vi "MyHostCode.vi"() -> ()   [LabVIEW 2012]
doc: "This VI was generated automatically using the FPGA Wizard. You can modify the VI normally."
uses:
  <vilib>/rvi/interface/nirviMethod/nirviMethod.xnode
  <vilib>/FPGAPlugInAG/Dynamic/niLvFpga_Run_Dynamic.vi
  <vilib>/rvi/interface/nirviCloseFPGA/nirviCloseFPGA.xnode
  <vilib>/rvi/interface/nirviOpenFPGA/nirviOpenFPGA.xnode
  <vilib>/FPGAPlugInAG/Dynamic/niLvFpga_Reset_Dynamic.vi
  MyFPGACode.vi
  <vilib>/rvi/interface/nirviReadWriteControl/nirviReadWriteControl.xnode
  <vilib>/rvi/errors/niLvFpgaAdjustHostInterfaceError.vi
  <vilib>/FPGAPlugInAG/Dynamic/niLvFpga_Close_Dynamic.vi
  NiFpgaLv.dll
  <vilib>/Utility/error.llb/Error Cluster From Error Code.vi
  <vilib>/rvi/interface/Simulation/niFpgaSimulationCallBeginRW.vi
panel:
  in  "PWM Settings (Port0/DIO5)":cluster{"ActiveTime":u32, "Period":u32}
  out "AI (ModA/AI0)":fxp<+/-,26,5> format="%.23g"
  in  "Local Stop 0":bool
  in  "Start 0":bool
  out "error out":errorcluster
  in  "Global Stop":bool
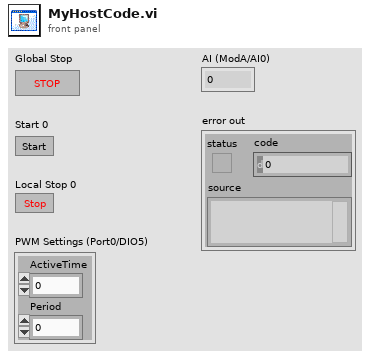
[diagram p1: front panel]
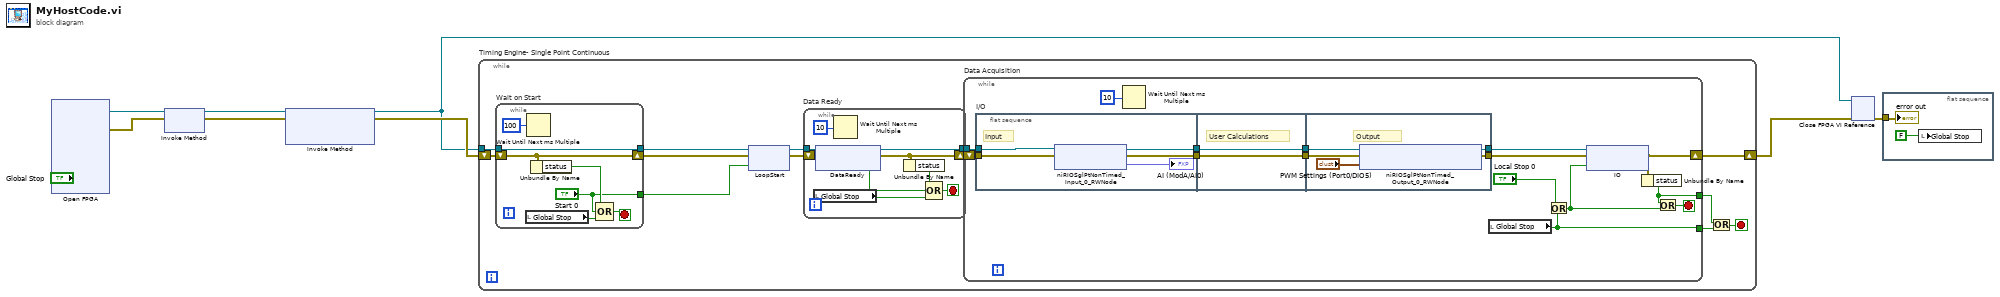
[diagram p0: block diagram]
diagram:
  n1 = xnode ("Open FPGA")() -> ("FPGA VI Reference Out"=w4:refnum<k20>, "error out"=w3:errorcluster)  [unwired: 2 in]
  n2 = xnode ("Invoke Method")("FPGA VI Reference In"=w4, "error in"=w3) -> ("FPGA VI Reference Out"=w7:refnum<k20>, "error out"=w8:errorcluster)
  n3 = xnode ("Invoke Method")("FPGA VI Reference In"=w7, "error in"=w8) -> ("FPGA VI Reference Out"=w5:refnum<k20>, "error out"=w6:errorcluster)  [unwired: 1 in]
  n4 = while "Timing Engine- Single Point Continuous" {
    tunnel: w5 -> [w20]
    shift-right: [w19] -> w2
    shift-left: w6 -> [w21]
    stop <- w14 stop-if-true
    n5 = while "Wait on Start" {
      tunnel: w20 -> [w36]
      tunnel: [w36] -> w11
      tunnel: ["Start 0"] -> w9
      shift-right: [w33] -> w10
      shift-left: w21 -> [w33]
      stop <- w37 stop-if-true
      n6 = local read "Global Stop"() -> (w34:bool)
      n7 = Wait Until Next ms Multiple(millisecond multiple=u32 100) -> ()  [unwired: 1 out]
      n8 = Unbundle By Name(w33) -> ("status"=w32:bool)
      n9 = Compound Arithmetic op=OR(w32, "Start 0", w34) -> (w37:bool)
    }
    n10 = xnode ("LoopStart")("FPGA VI Reference In"=w11, "error in"=w10, "Start 0"=w9) -> ("FPGA VI Reference Out"=w18:refnum<k20>, "error out"=w16:errorcluster)
    n11 = while "Data Ready" {
      tunnel: w18 -> [w30]
      tunnel: [w29] -> w17
      shift-right: [w23] -> w12
      shift-left: w16 -> [w28]
      stop <- w24 stop-if-true
      n12 = local read "Global Stop"() -> (w26:bool)
      n13 = xnode ("DataReady")("FPGA VI Reference In"=w30, "error in"=w28) -> ("FPGA VI Reference Out"=w29:refnum<k20>, "error out"=w23:errorcluster, "Data Ready 0"=w25:bool)
      n14 = Wait Until Next ms Multiple(millisecond multiple=u32 10) -> ()  [unwired: 1 out]
      n15 = Unbundle By Name(w23) -> ("status"=w22:bool)
      n16 = Compound Arithmetic op=OR(w22, w25, w26) -> (w24:bool)
    }
    n17 = while "Data Acquisition" {
      tunnel: w17 -> [w41]
      tunnel: [w43] -> w15
      tunnel: [w42] -> w13
      shift-right: [w44] -> w19
      shift-left: w12 -> [w40]
      stop <- w52 stop-if-true
      n18 = flat-sequence "I/O" {
        tunnel: w41 -> [w55]
        tunnel: [w56] -> w50
        tunnel: [w54] -> w47
        tunnel: w40 -> [w57]
        tunnel: w50 -> [w59]
        tunnel: [w59] -> w49
        tunnel: [w58] -> w48
        tunnel: w47 -> [w58]
        tunnel: [w63] -> w46
        tunnel: [w61] -> w45
        tunnel: w49 -> [w64]
        tunnel: w48 -> [w62]
        frame #0 {
          # "Input"
          n19 = xnode ("niRIOSglPtNonTimed_Input_0_RWNode")("FPGA VI Reference In"=w55, "error in"=w57) -> ("FPGA VI Reference Out"=w54:refnum<k20>, "error out"=w56:errorcluster, "AI (ModA/AI0)"=→"AI (ModA/AI0)":fxp<+/-,26,5>)
        }
        frame #1 {
          # "User Calculations"
        }
        frame #2 {
          # "Output"
          n20 = xnode ("niRIOSglPtNonTimed_Output_0_RWNode")("FPGA VI Reference In"=w62, "error in"=w64, "PWM Settings (Port0/DIO5)"="PWM Settings (Port0/DIO5)") -> ("FPGA VI Reference Out"=w61:refnum<k20>, "error out"=w63:errorcluster)
        }
      }
      n21 = Wait Until Next ms Multiple(millisecond multiple=u32 10) -> ()  [unwired: 1 out]
      n22 = local read "Global Stop"() -> (w43:bool)
      n23 = Or(x="Local Stop 0", y=w43) -> (x .or. y?=w38:bool)
      n24 = xnode ("IO")("FPGA VI Reference In"=w45, "error in"=w46, "Local Stop 0"=w38) -> ("error out"=w44:errorcluster)  [unwired: 1 out]
      n25 = Unbundle By Name(w44) -> ("status"=w42:bool)
      n26 = Or(x=w42, y=w38) -> (x .or. y?=w52:bool)
    }
    n27 = Or(x=w13, y=w15) -> (x .or. y?=w14:bool)
  }
  n28 = xnode ("Close FPGA VI Reference")("FPGA VI Reference In"=w5, "error in"=w2) -> ("error out"=w1:errorcluster)
  n29 = flat-sequence {
    tunnel: w1 -> [w66]
    frame #0 {
      n30 = local write "Global Stop"(FALSE ("Global Stop")) -> ()
      "error out" <- w66
    }
  }
